vi "Send Boolean.vi"(6 "Name (Use Control Label)":string, 7 "Message Priority (Normal)":T1=enum."Normal", 8 "error in (no error)":errorcluster, 9 "Value":bool, 10 "Bool Refnum":refnum<vi>, 11 "Message Enqueuer in":refnum<class "Message Enqueuer.lvclass">) -> (0 "error out":errorcluster)   [LabVIEW 2015, in "Broadcast Boolean Msg.lvclass"]
uses:
  Broadcast Boolean Msg.lvclass
  <vilib>/ActorFramework/Message Enqueuer/Message Enqueuer.lvclass
  <vilib>/ActorFramework/Message Enqueuer/Message Priority.ctl
  Broadcast Boolean Msg.lvclass/Broadcast Boolean Msg.ctl
  <vilib>/ActorFramework/Message Enqueuer/Message Enqueuer.lvclass/Message Enqueuer.ctl
  <vilib>/ActorFramework/Message Priority Queue/Priority Enqueue.vi
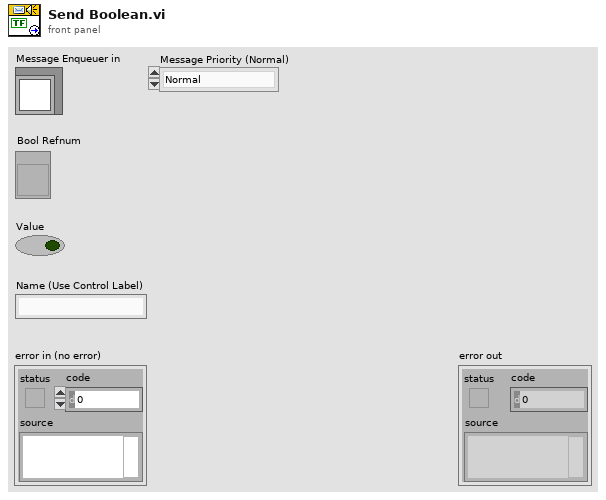
[diagram p1: front panel]
types:
  T1 = typedef "Actor Framework.lvlib/Message Enqueuer.lvclass/Message Priority.ctl" = enum16{"Low", "Normal", "High"}
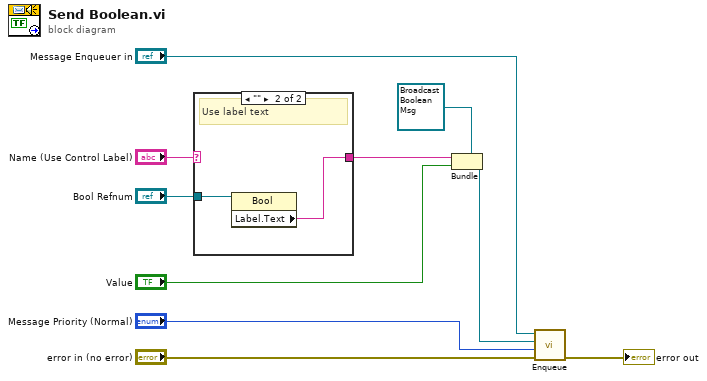
[diagram p0: block diagram]
diagram:
  n1 = case shown="\"\"" "Name (Use Control Label)" {
    selector: "Name (Use Control Label)" -> [w11 _]
    tunnel: [w11 w12] -> w3
    tunnel: "Bool Refnum" -> [_ w13]
    frame Default {
      # "Use string provided"
    }
    frame "" {
      # "Use label text"
      n2 = property class="Bool"(reference=w13) -> ("Label.Text"=w12:string)  [unwired: 1 in, 2 out]
    }
  }
  n3 = Bundle(cluster=refnum<class "Broadcast Boolean Msg.lvclass"> refnum ("Broadcast Boolean Msg in"), w3, "Value") -> (w7:refnum<class "Broadcast Boolean Msg.lvclass">)
  n4 = call <vilib>:"Enqueue.vi"("error in (no error)"="error in (no error)", "Message Priority (Normal)"="Message Priority (Normal)", "Message"=w7, "Message Enqueuer in"="Message Enqueuer in") -> ("error out"=→"error out":errorcluster)  [unwired: 6 in, 1 out]
